vi "Control_MoveSnakeTail.vi"(2 "AddGrowthCycles":i8, 6 "InitialDirection":T2, 8 "InitialPosition":i16, 9 "Reset":bool, 10 "Player":T1) -> (16 "Growing?":bool)   [LabVIEW 2018]
uses:
  TypDefs/Direction_Enum.ctl
  TypDefs/Player_Enum.ctl
  TypDefs/Tile_Enum.ctl
  <vilib>/rvi/DataTransferAndStorage/Container/Common/niFpgaContainerExecOnDevCompGetState.vi
  <vilib>/rvi/Emulation/niFpgaEmulationIsFPGAContextNoSignature.vi
  <vilib>/rvi/DataTransferAndStorage/Container/Common/niFpgaContainerGetUniqueNameForEmu.vi
  <vilib>/rvi/Emulation/niFpgaProcessEmulError.vi
  <vilib>/rvi/Emulation/niFpgaSctlEmulationGetInTimedLoop.vi
  <vilib>/rvi/errors/nirviReportUnexpectedCaseInternalError (U32).vi
  <vilib>/rvi/Memory/Memory_Emulation/niFpgaMemoryEmulationCacheClearOnFirstRun.vi
  <vilib>/rvi/Memory/Memory_Emulation/nirvimemoryEmulationManagerCache_MakeExclusive.vi
  <vilib>/rvi/Memory/Memory_Emulation/niFpgaMemoryEmulationValidateCache.vi
  <vilib>/rvi/Memory/Memory_Emulation/nirvimemoryEmulationManagerCache_InsertValue.vi
  <vilib>/Utility/error.llb/Clear Errors.vi
  <vilib>/rvi/Memory/Memory_Emulation/nirvimemoryEmulationManagerCache_ReleaseExclusive.vi
  <vilib>/rvi/Memory/Memory_Emulation/nirvimemoryEmulationManagerCache_GetValue.vi
  <vilib>/rvi/Memory/Memory_Emulation/nirvimemoryEmulationManagerCache_SetValue.vi
  <vilib>/rvi/Emulation/niFpgaSctlEmulationResourceMgr.vi
  <vilib>/rvi/DataTransferAndStorage/Container/XNode/niFpgaContainer.xnode
  <vilib>/rvi/Memory/Memory_Emulation/niFpgaMemoryEmulationRefIn.vi
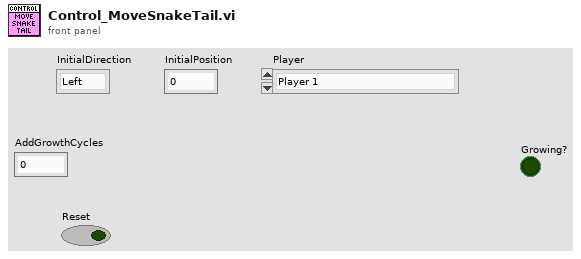
[diagram p1: front panel]
types:
  T1 = typedef "Player_Enum.ctl" = enum16{"Player 1", "Player 2"}
  T2 = typedef "Direction_Enum.ctl" = enum8{"Left", "Right", "Up", "Down"}
  T3 = typedef "Tile_Enum.ctl" = enum8{"Empty", "Snake1_HeadPointingUp", "Snake1_HeadPointingDown", "Snake1_HeadPointingLeft", "Snake1_HeadPointingRight", "Snake1_DeadPointingUp", "Snake1_DeadPointingDown", "Snake1_DeadPointingLeft", "Snake1_DeadPointingRight", "Snake1_TailPointingUp", "Snake1_TailPointingDown", "Snake1_TailPointingLeft", "Snake1_TailPointingRight", "Snake1_Horizontal", "Snake1_Vertical", "Snake1_UpperLeftCorner", "Snake1_UpperRightCorner", "Snake1_LowerLeftCorner", "Snake1_LowerRightCorner", "Snake2_HeadPointingUp", "Snake2_HeadPointingDown", "Snake2_HeadPointingLeft", "Snake2_HeadPointingRight", "Snake2_DeadPointingUp", "Snake2_DeadPointingDown", "Snake2_DeadPointingLeft", "Snake2_DeadPointingRight", "Snake2_TailPointingUp", "Snake2_TailPointingDown", "Snake2_TailPointingLeft", "Snake2_TailPointingRight", "Snake2_Horizontal", "Snake2_Vertical", "Snake2_UpperLeftCorner", "Snake2_UpperRightCorner", "Snake2_LowerLeftCorner", "Snake2_LowerRightCorner", "Wall_Horizontal", "Wall_Vertical", "Wall_UpperLeftCorner", "Wall_UpperRightCorner", "Wall_LowerLeftCorner", "Wall_LowerRightCorner", "Pickup_SpeedUp", "Pickup_Stop", "Pickup_Item1", "Pickup_Item2", "Pickup_Item3", "Pickup_Item4", "Pickup_Item5", "Pickup_Item6"}
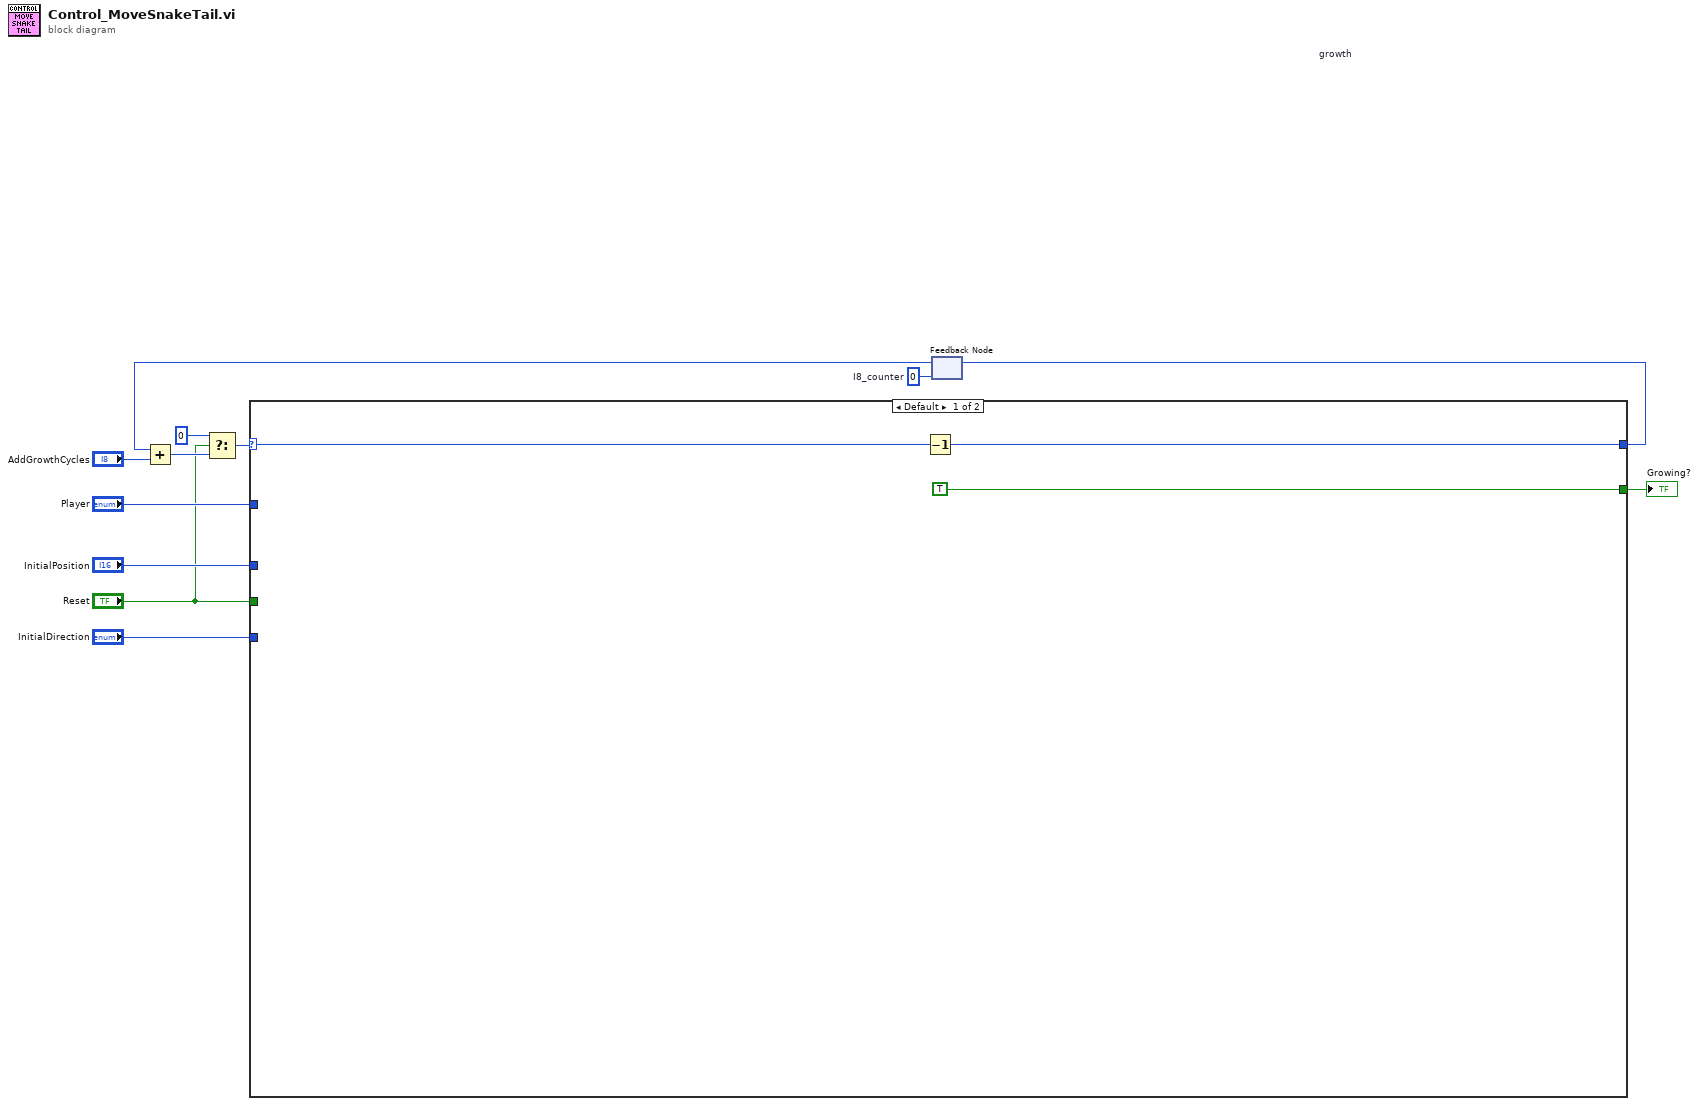
[diagram p0: block diagram]
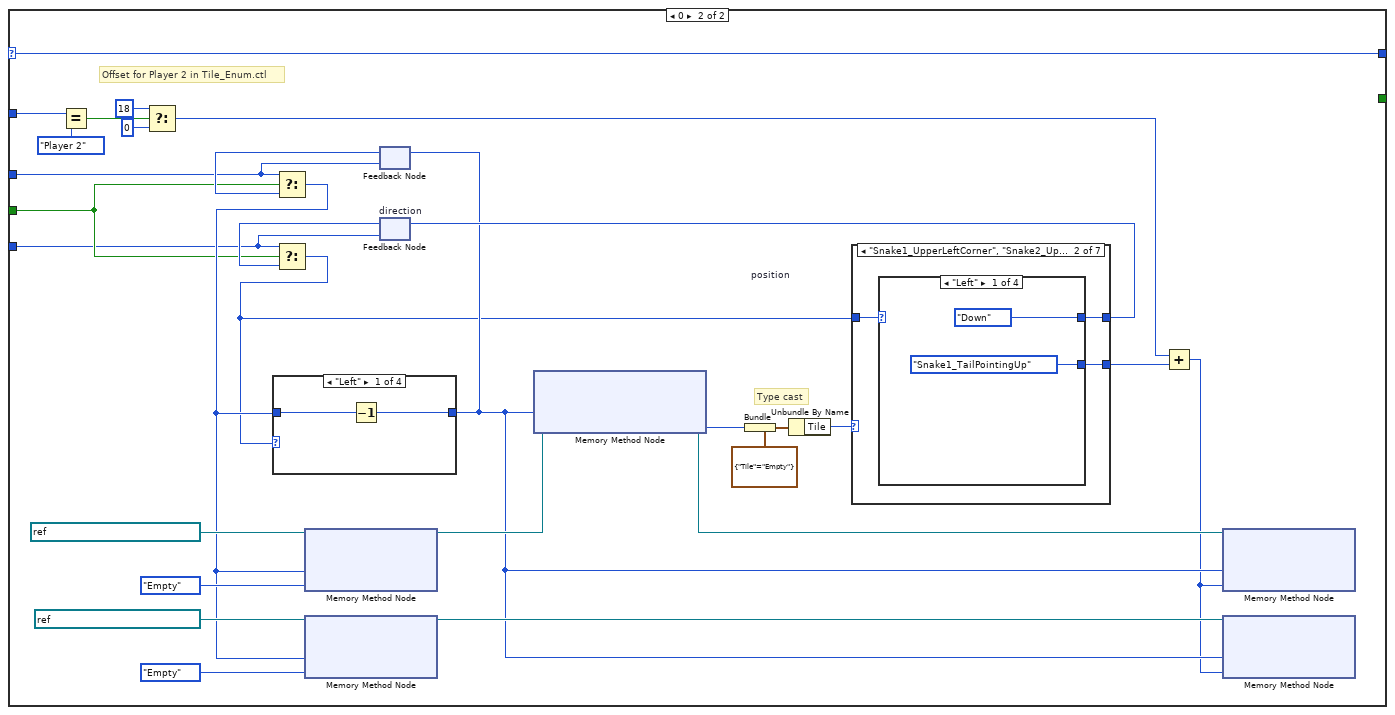
[diagram p2: hidden frame]
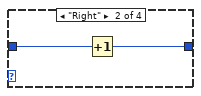
[diagram p3: hidden frame]
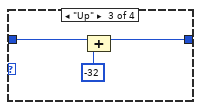
[diagram p4: hidden frame]
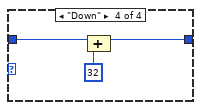
[diagram p5: hidden frame]
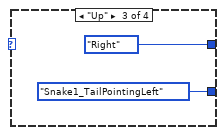
[diagram p8: hidden frame]
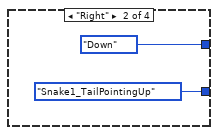
[diagram p11: hidden frame]
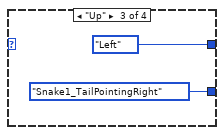
[diagram p12: hidden frame]
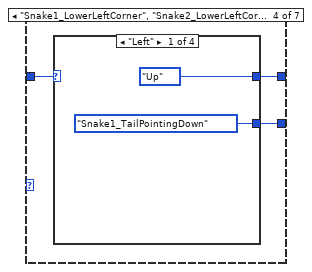
[diagram p14: hidden frame]
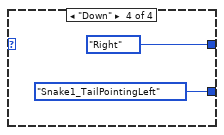
[diagram p17: hidden frame]
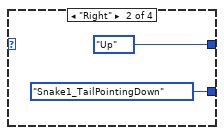
[diagram p19: hidden frame]
diagram:
  w10 = i8 0  # I8_counter
  n1 = feedback #1 "growth"(w10) -> (w8:i8)
  n2 = Add(x=w8, y="AddGrowthCycles") -> (x+y=w5:i8)
  n3 = Select(t=i8 0, s="Reset", f=w5) -> (s? t:f=w4:i8)
  n4 = case shown="Default" w4 {
    selector: w4 -> [w15 w39]
    tunnel: "InitialDirection" -> [_ w16]
    tunnel: "InitialPosition" -> [_ w17]
    tunnel: [w14 w39] -> w9
    tunnel: "Player" -> [_ w24]
    tunnel: "Reset" -> [_ w18]
    tunnel: [TRUE _] -> w1
    frame Default {
      n5 = Decrement(x=w15) -> (x-1=w14:i8)
    }
    frame 0 {
      # "Offset for Player 2 in Tile_Enum.ctl"
      # "Type cast"
      n6 = Equal?(x=w24, y=Player_Enum."Player 2") -> (x = y?=w27:bool)
      n7 = Select(t=u8 18, s=w27, f=u8 0) -> (s? t:f=w23:u8)
      n8 = feedback #2 "position"(w17) -> (w22:i16)
      n9 = Select(t=w17, s=w18, f=w22) -> (s? t:f=w21:i16)
      n10 = xnode ("Memory Method Node")("Address"=w21, "Data"=Tile_Enum."Empty" ("Tile"), "Memory In"=refnum<k21> "BlockMem_SlowGameMap") -> ("Memory Out"=w44:refnum<k21>)
      n11 = xnode ("Memory Method Node")("Address"=w21, "Data"=Tile_Enum."Empty" ("Tile"), "Memory In"=refnum<k21> "BlockMem_FastGameMap") -> ("Memory Out"=w33:refnum<k21>)
      n12 = feedback #3 "direction"(w16) -> (w20:T2)
      n13 = Select(t=w16, s=w18, f=w20) -> (s? t:f=w19:T2)
      n14 = case shown="\"Left\"" w19 {
        tunnel: [w46 w48 w50 w53] -> w32
        tunnel: w21 -> [w45 w47 w49 w52]
        frame "Left" {
          n15 = Decrement(x=w45) -> (x-1=w46:i16)
        }
        frame "Right" {
          n16 = Increment(x=w47) -> (x+1=w48:i16)
        }
        frame "Up" {
          n17 = Compound Arithmetic op=ADD(w49, i16 -32 ("y")) -> (w50:i16)
        }
        frame "Down" {
          n18 = Compound Arithmetic op=ADD(w52, i16 32 ("y")) -> (w53:i16)
        }
      }
      n19 = feedback-in #2(w32) -> ()
      n20 = xnode ("Memory Method Node")("Address"=w32, "Memory In"=w44) -> ("Data"=w37:u8, "Memory Out"=w43:refnum<k21>)
      n21 = Bundle(cluster=cluster{"Tile":T3} {"Tile"=enum."Empty"}, "Tile"=w37) -> (w41:cluster{"Tile":T3})
      n22 = Unbundle By Name(w41) -> ("Tile"=w40:T3)
      n23 = case shown="\"Snake1_UpperLeftCorner\", \"Snake2_UpperLeftCorner\"" w40 {
        tunnel: [w55 w58 w65 w72 w79 w86 w93] -> w38
        tunnel: w19 -> [w55 w57 w64 w71 w78 w85 w92]
        tunnel: [_ w56 w63 w70 w77 w84 w91] -> w30
        frame Default {
          # "Should never execute"
        }
        frame "Snake1_UpperLeftCorner", "Snake2_UpperLeftCorner" {
          n24 = case shown="\"Left\"" w57 {
            tunnel: [Direction_Enum."Down" ("initial_direction") _ Direction_Enum."Right" ("initial_direction") _] -> w58
            tunnel: [Tile_Enum."Snake1_TailPointingUp" ("Tile") _ Tile_Enum."Snake1_TailPointingLeft" ("Tile") _] -> w56
            frame "Left" {
            }
            frame "Right" {
            }
            frame "Up" {
            }
            frame "Down" {
            }
          }
        }
        frame "Snake1_UpperRightCorner", "Snake2_UpperRightCorner" {
          n25 = case shown="\"Left\"" w64 {
            tunnel: [_ Direction_Enum."Down" ("initial_direction") Direction_Enum."Left" ("initial_direction") _] -> w65
            tunnel: [_ Tile_Enum."Snake1_TailPointingUp" ("Tile") Tile_Enum."Snake1_TailPointingRight" ("Tile") _] -> w63
            frame "Left" {
            }
            frame "Right" {
            }
            frame "Up" {
            }
            frame "Down" {
            }
          }
        }
        frame "Snake1_LowerLeftCorner", "Snake2_LowerLeftCorner" {
          n26 = case shown="\"Left\"" w71 {
            tunnel: [Direction_Enum."Up" ("initial_direction") _ _ Direction_Enum."Right" ("initial_direction")] -> w72
            tunnel: [Tile_Enum."Snake1_TailPointingDown" ("Tile") _ _ Tile_Enum."Snake1_TailPointingLeft" ("Tile")] -> w70
            frame "Left" {
            }
            frame "Right" {
            }
            frame "Up" {
            }
            frame "Down" {
            }
          }
        }
        frame "Snake1_LowerRightCorner", "Snake2_LowerRightCorner" {
          n27 = case shown="\"Left\"" w78 {
            tunnel: [_ Direction_Enum."Up" ("initial_direction") _ Direction_Enum."Left" ("initial_direction")] -> w79
            tunnel: [_ Tile_Enum."Snake1_TailPointingDown" ("Tile") _ Tile_Enum."Snake1_TailPointingRight" ("Tile")] -> w77
            frame "Left" {
            }
            frame "Right" {
            }
            frame "Up" {
            }
            frame "Down" {
            }
          }
        }
        frame "Snake1_Horizontal", "Snake2_Horizontal" {
          n28 = case shown="\"Left\"" w85 {
            selector: w85 -> [w88 w89 _ _]
            tunnel: [w88 w89 _ _] -> w86
            tunnel: [Tile_Enum."Snake1_TailPointingRight" ("Tile") Tile_Enum."Snake1_TailPointingLeft" ("Tile") _ _] -> w84
            frame "Left" {
            }
            frame "Right" {
            }
            frame "Up" {
            }
            frame "Down" {
            }
          }
        }
        frame "Snake1_Vertical", "Snake2_Vertical" {
          n29 = case shown="\"Left\"" w92 {
            selector: w92 -> [_ _ w95 w97]
            tunnel: [_ _ w95 w97] -> w93
            tunnel: [_ _ Tile_Enum."Snake1_TailPointingDown" ("Tile") Tile_Enum."Snake1_TailPointingUp" ("Tile")] -> w91
            frame "Left" {
            }
            frame "Right" {
            }
            frame "Up" {
            }
            frame "Down" {
            }
          }
        }
      }
      n30 = feedback-in #3(w38) -> ()
      n31 = Add(x=w23, y=w30) -> (x+y=w29:u8)
      n32 = xnode ("Memory Method Node")("Address"=w32, "Data"=w29, "Memory In"=w43) -> ()  [unwired: 1 out]
      n33 = xnode ("Memory Method Node")("Address"=w32, "Data"=w29, "Memory In"=w33) -> ()  [unwired: 1 out]
    }
  }
  "Growing?" <- w1
  n34 = feedback-in #1(w9) -> ()
